vi "Global Constants.vi"() -> ()   [LabVIEW 2019]
uses:
  TypeDefs/Constants.ctl
panel:
  out "constants":T1
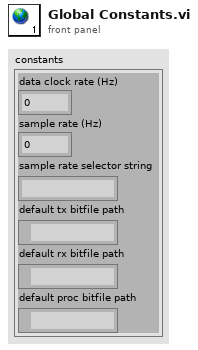
[diagram p1: front panel]
types:
  T1 = typedef "Constants.ctl" = cluster{"data clock rate (Hz)":dbl, "sample rate (Hz)":dbl, "sample rate selector string":string, "default tx bitfile path":path, "default rx bitfile path":path, "default proc bitfile path":path}
diagram:
